vi "square waveform.vi"() -> ()   [LabVIEW 2019]
uses:
  <vilib>/measure/mamon.llb/Trigger Detection for 1 Channel.vi
  <vilib>/measure/NI_MABase.lvlib
  <vilib>/measure/NI_MAPro.lvlib
panel:
  out "In Range?":bool
  out "Elapsed Time (s) 2":dbl caption="Elapsed Time (s)"
  out "x > y?":bool
  in  "Time Target (s)":dbl=5.0 format="%#_13g"
  out "Elapsed Time (s)":dbl
  out "Time has Elapsed":bool
  in  "Reset":bool
  in  "sampling info":cluster{"Fs":dbl, "#s":dbl}={"Fs"=1000.0, "#s"=1000.0} {"Fs" format="%.2p"}
  out "Pulse Trend":waveform(i16)(graph) caption="Waveform Chart - Dark"
  in  "duty cycle (%)":dbl=50.0 format="%0.2f"
  in  "amplitude":dbl=1.0 format="%0.2p"
  in  "frequency":dbl=10.0 format="%0.2p"
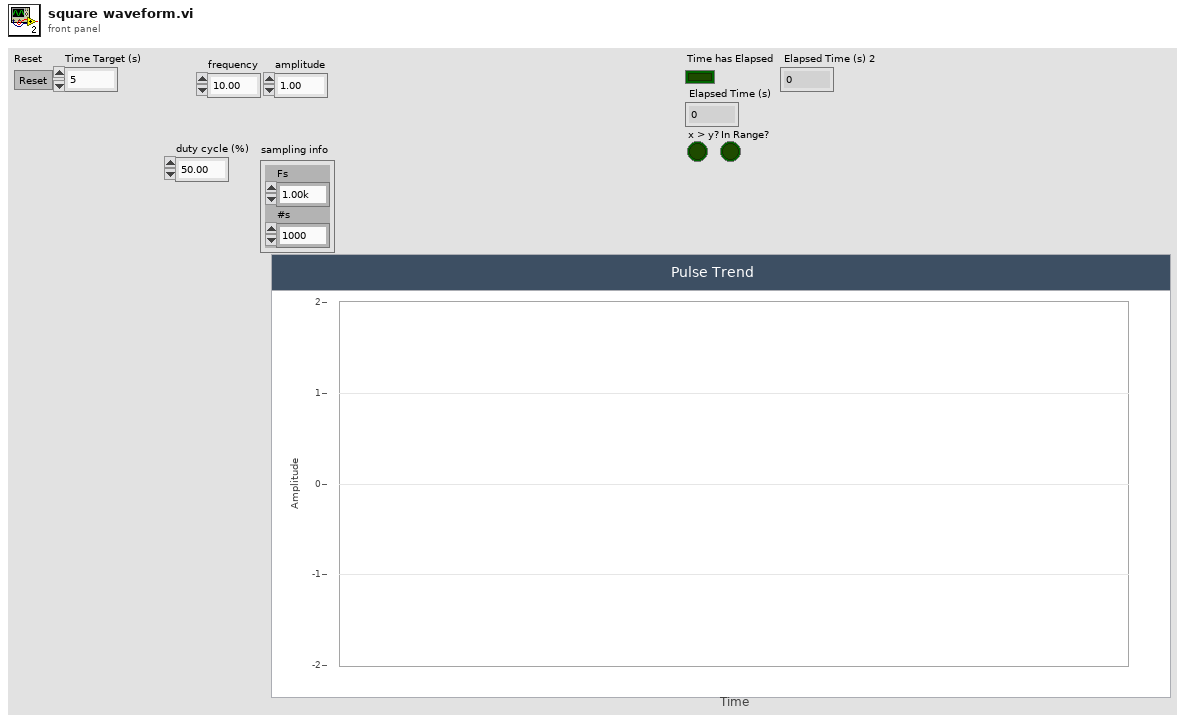
[diagram p1: front panel]
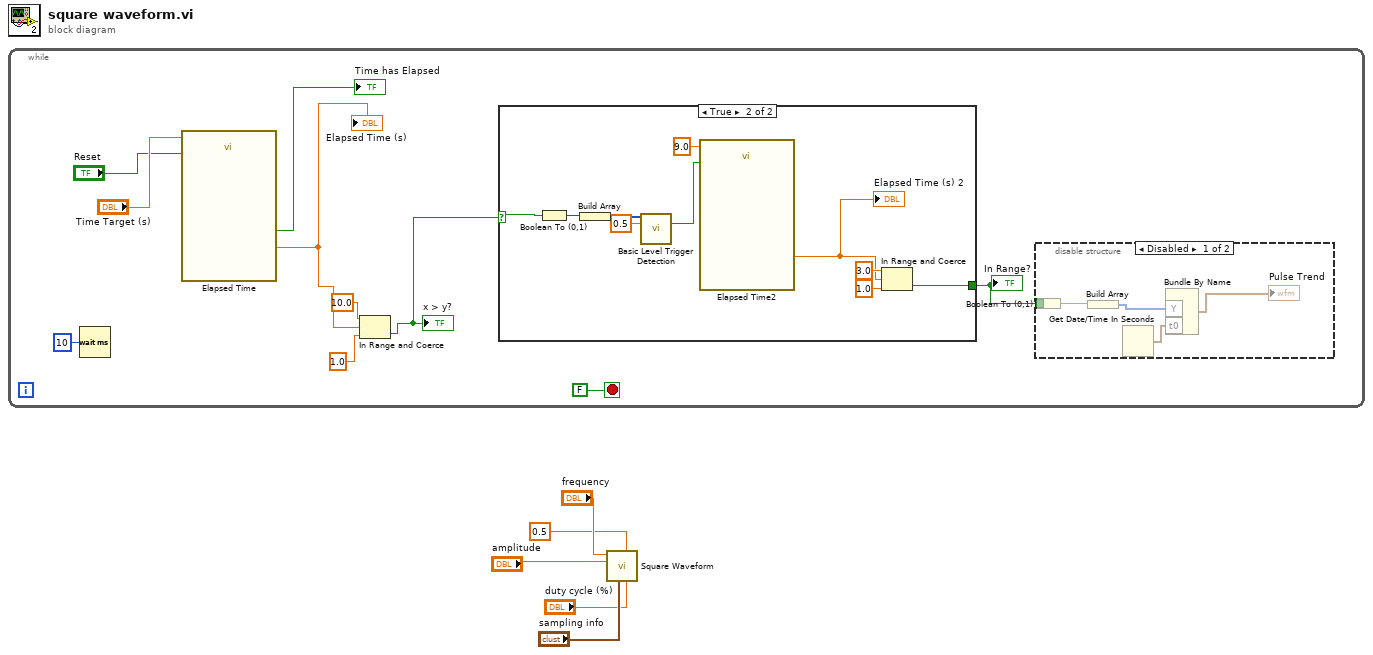
[diagram p0: block diagram]
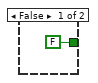
[diagram p3: hidden frame]
diagram:
  n1 = while {
    stop <- FALSE stop-if-true
    n2 = Wait (ms)(milliseconds to wait=u32 10 ("millisecond multiple")) -> ()  [unwired: 1 out]
    n3 = call "Elapsed Time"("Time Target (s)"="Time Target (s)", "Reset"="Reset") -> ("Elapsed Time (s)"=w10:dbl, "Time has Elapsed"=→"Time has Elapsed":bool)  [unwired: 10 in, 6 out]
    "Elapsed Time (s)" <- w10
    n4 = In Range and Coerce(upper limit=10.0, x=w10, lower limit=1.0) -> (In Range?=w7:bool)  [unwired: 1 out]
    "x > y?" <- w7
    n5 = case shown="True" w7 {
      selector: w7 -> [_ w28]
      tunnel: [FALSE w22] -> w6
      frame False {
      }
      frame True {
        n6 = Boolean To (0,1)(Boolean=w28) -> (0, 1=w27:i16)
        n7 = Build Array(w27) -> (w26:i16[])
        n8 = call-poly <vilib>:"Basic Level Trigger Detection.vi"("signal in"=w26, "level"=0.5) -> ("trigger detected?"=w24:bool)  [unwired: 11 in, 2 out]
        n9 = call "Elapsed Time2"("Time Target (s)"=9.0, "Reset"=w24) -> ("Elapsed Time (s)"=w23:dbl)  [unwired: 10 in, 7 out]
        "Elapsed Time (s) 2" <- w23
        n10 = In Range and Coerce(upper limit=3.0, x=w23, lower limit=1.0) -> (In Range?=w22:bool)  [unwired: 1 out]
      }
    }
    "In Range?" <- w6
    n11 = disable-structure shown="Disabled" {
      disable-tunnel: w6 -> [w20 _]
      frame Disabled {
        n12 = Boolean To (0,1)(Boolean=w20) -> (0, 1=w19:i16)
        n13 = Build Array(w19) -> (w18:i16[])
        n14 = Get Date/Time In Seconds() -> (seconds since 1Jan1904=w17:timestamp)
        n15 = Bundle By Name("Y"=w18, "t0"=w17) -> (→"Pulse Trend":waveform(i16))  [unwired: 1 in]
      }
      frame Enabled {
      }
    }
  }
  n16 = call <vilib>:"Square Waveform.vi"("duty cycle (%)"="duty cycle (%)", "offset"=0.5, "sampling info"="sampling info", "amplitude"="amplitude", "frequency"="frequency") -> ()  [unwired: 5 in, 2 out]
